vi "Add Index.vi"(8 "Count":i32, 10 "Byte":u8, 11 "Indices Input":i32[](array[numeric])) -> (0 "Count+1":i32, 3 "Indices Output":i32[](array[numeric]))   [LabVIEW 2011]
uses:
  GlobalVariables.vi
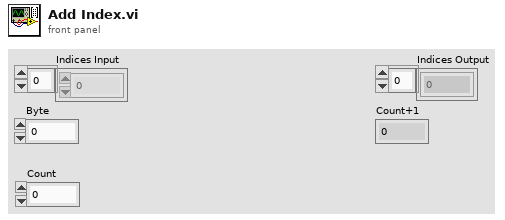
[diagram p1: front panel]
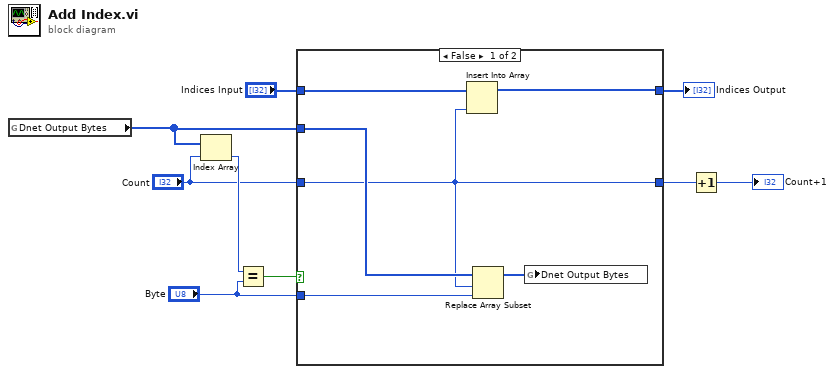
[diagram p0: block diagram]
diagram:
  n1 = global read "GlobalVariables.vi" "Dnet Output Bytes"() -> (w9:u8[])
  n2 = Index Array(array=w9, index="Count") -> (element=w7:u8)
  n3 = Equal?(x=w7, y="Byte") -> (x = y?=w8:bool)
  n4 = case shown="False" w8 {
    tunnel: w9 -> [w14 _]
    tunnel: "Indices Input" -> [w13 w17]
    tunnel: [w12 w17] -> w5
    tunnel: "Byte" -> [w11 _]
    tunnel: "Count" -> [w10 w16]
    tunnel: [w10 w16] -> w2
    frame False {
      n5 = Insert Into Array(array=w13, new element=w10) -> (w12:i32[])  [unwired: 1 in]
      n6 = Replace Array Subset(array=w14, new element=w11, index=w10) -> (w15:u8[])
      n7 = global write "GlobalVariables.vi" "Dnet Output Bytes"(w15) -> ()
    }
    frame True {
    }
  }
  "Indices Output" <- w5
  n8 = Increment(x=w2) -> (x+1=→"Count+1":i32)
